vi "Untitled 2.vi"() -> ()   [LabVIEW 2021]
panel:
  out "XY Graph":cluster{"Y":dbl[], "Y":dbl[]}[](graph)
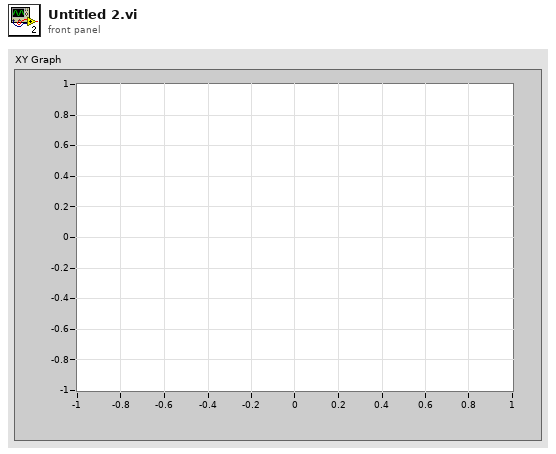
[diagram p1: front panel]
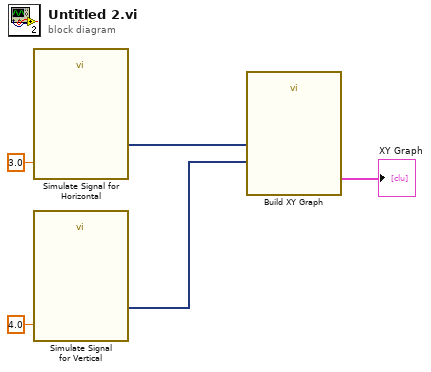
[diagram p0: block diagram]
diagram:
  n1 = call "Simulate Signal for Horizontal"("Frequency"=3.0) -> ("Sine"=w3:dynamicdata)  [unwired: 5 in, 9 out]
  n2 = call "Simulate Signal\nfor Vertical"("Frequency"=4.0) -> ("Sine"=w4:dynamicdata)  [unwired: 5 in, 9 out]
  n3 = call "Build XY Graph"("Y Input"=w4, "X Input"=w3) -> ("XY Graph"=→"XY Graph":cluster{"Y":dbl[], "Y":dbl[]}[])  [unwired: 3 in, 6 out]
